vi "Read DAQmx Config.vi"(8 "error in (no error)":errorcluster, 10 "DAQmxChannel":T1, 11 "configuration file path":path) -> (0 "error out":errorcluster, 2 "DAQmx Channel out":T1, 3 "configuration file path out":path)   [LabVIEW 2018]
doc: "Odczytuje z pliku ustawienia akwizycji dla karty DAQ"
uses:
  controls/Daqtypedef.ctl
  <vilib>/Utility/config.llb/NI_LVConfig.lvlib
  <userlib>/_OpenG.lib/variantconfig/variantconfig.llb/openg_variant_configuration_file.lvlib
  <userlib>/_OpenG.lib/error/error.llb/openg_error.lvlib
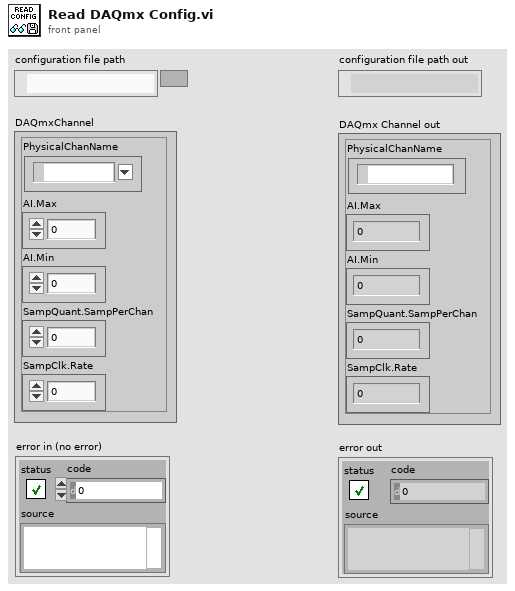
[diagram p1: front panel]
types:
  T1 = typedef "Daqtypedef.ctl" = cluster{"PhysicalChanName":tag, "AI.Max":dbl, "AI.Min":dbl, "SampQuant.SampPerChan":i32, "SampClk.Rate":dbl}
  T2 = typedef "NI_LVConfig.lvlib/Config Data RefNum.ctl" = refnum<k1>
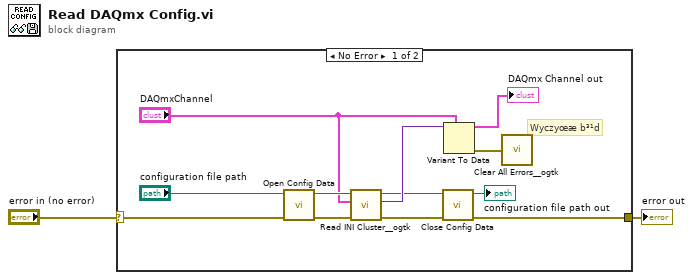
[diagram p0: block diagram]
diagram:
  n1 = case shown="No Error" "error in (no error)" {
    selector: "error in (no error)" -> [w5 w15]
    tunnel: [w8 w15] -> w2
    frame No Error {
      # "Wyczyœæ b³¹d"
      n2 = call <vilib>:"Open Config Data.vi"("error in (no error)"=w5, "configuration file path"="configuration file path") -> ("error out"=w14:errorcluster, "refnum"=w12:T2)  [unwired: 7 in, 1 out]
      n3 = call <userlib>:"Read INI Cluster__ogtk.vi"("error in (no error)"=w14, "INI Fomatted Cluster Type"="DAQmxChannel", "refnum"=w12) -> ("error out"=w10:errorcluster, "INI Fomatted Cluster"=w11:variant, "dup refnum"=w9:T2)  [unwired: 4 in, 2 out]
      n4 = call <vilib>:"Close Config Data.vi"("error in (no error)"=w10, "refnum"=w9) -> ("error out"=w8:errorcluster, "file path"=→"configuration file path out":path)  [unwired: 8 in]
      n5 = Variant To Data(type="DAQmxChannel", Variant=w11) -> (data=→"DAQmx Channel out":T1, error out=w3:errorcluster)  [unwired: 1 in]
      n6 = call <userlib>:"Clear All Errors__ogtk.vi"("Upsteam Error (optional)"=w3, "Error In"=w3) -> ()  [unwired: 2 in, 1 out]
    }
    frame Error {
    }
  }
  "error out" <- w2
